vi "test shutter.vi"() -> ()   [LabVIEW 2015]
uses:
  <vilib>/ActorFramework/Actor/Actor.lvclass
  Hardware/Uniblitz Shutter/Uniblitz Shutter.lvclass
  Type Defs/Excitation.ctl
  Type Defs/Shutter Configuration.ctl
  Hardware/Uniblitz Shutter Messages/Open Shutter Msg/Open Shutter Msg.lvclass
  Hardware/Uniblitz Shutter Messages/Close Shutter Msg/Close Shutter Msg.lvclass
  <vilib>/ActorFramework/Stop Msg/Stop Msg.lvclass
panel:
  in  "Boolean":bool
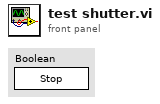
[diagram p1: front panel]
types:
  T1 = typedef "Shutter Configuration.ctl" = cluster{"Excitation":T2, "IO Line":tag}
  T2 = typedef "Excitation.ctl" = enum16{"Cy2 (473 nm)", "Cy3 (532 nm)", "Cy5 (639 nm)", "Cy7 (730 nm)"}
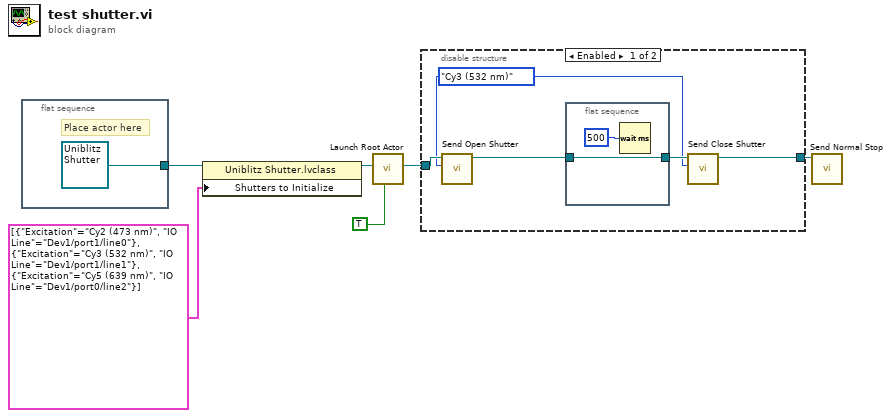
[diagram p0: block diagram]
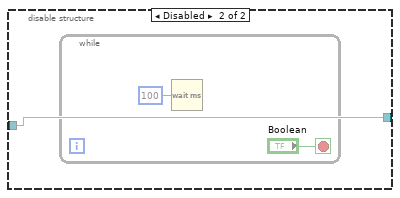
[diagram p2: hidden frame]
diagram:
  n1 = flat-sequence {
    tunnel: [refnum<class "Uniblitz Shutter.lvclass"> refnum ("Uniblitz Shutter.lvlib:Uniblitz Shutter.lvclass")] -> w6
    frame #0 {
      # "Place actor here"
    }
  }
  n2 = property class="Uniblitz Shutter.lvclass"(reference=w6, "Shutters to Initialize"=T1[] [{"Excitation"=enum."Cy2 (473 nm)", "IO Line"="Dev1/port1/line0"}, {"Excitation"=enum."Cy3 (532 nm)", "IO Line"="Dev1/port1/line1"}, {"Excitation"=enum."Cy5 (639 nm)", "IO Line"="Dev1/port0/line2"}]) -> (reference out=w5:refnum<class "Uniblitz Shutter.lvclass">)  [unwired: 1 in, 1 out]
  n3 = call <vilib>:"Launch Root Actor.vi"("Open Actor Core front panel? (F)"=TRUE, "Actor"=w5) -> ("Actor's Enqueuer"=w3:refnum<class "Message Enqueuer.lvclass">)  [unwired: 8 in, 1 out]
  n4 = disable-structure shown="Enabled" {
    disable-tunnel: w3 -> [w12 w15]
    disable-tunnel: [w8 w15] -> w2
    frame Enabled {
      w9 = Excitation."Cy3 (532 nm)" ("Shutter to Open")
      n5 = call "Send Open Shutter.vi"("Shutter to Open"=w9, "Message Enqueuer"=w12) -> ("Message Enqueuer out"=w11:refnum<class "Message Enqueuer.lvclass">)  [unwired: 8 in, 1 out]
      n6 = flat-sequence {
        tunnel: w11 -> [w14]
        tunnel: [w14] -> w10
        frame #0 {
          n7 = Wait (ms)(milliseconds to wait=u32 500) -> ()  [unwired: 1 out]
        }
      }
      n8 = call "Send Close Shutter.vi"("Shutter to Close"=w9, "Message Enqueuer"=w10) -> ("Message Enqueuer out"=w8:refnum<class "Message Enqueuer.lvclass">)  [unwired: 8 in, 1 out]
    }
    frame Disabled {
      n9 = while {
        stop <- "Boolean" stop-if-true
        n10 = Wait (ms)(milliseconds to wait=u32 100) -> ()  [unwired: 1 out]
      }
    }
  }
  n11 = call <vilib>:"Send Normal Stop.vi"("Message Enqueuer"=w2) -> ()  [unwired: 10 in, 1 out]
